vi "Remove Value.vi"(8 "error in (no error)":errorcluster, 10 "Name":string, 11 "Session in":refnum<class "Session.lvclass">) -> (0 "error out":errorcluster, 1 "Found?":bool, 2 "Removed Value":string, 3 "Session out":refnum<class "Session.lvclass">)   [LabVIEW 2020, in "HTTP Server.lvlib" / "Session.lvclass"]
uses:
  Session.lvclass
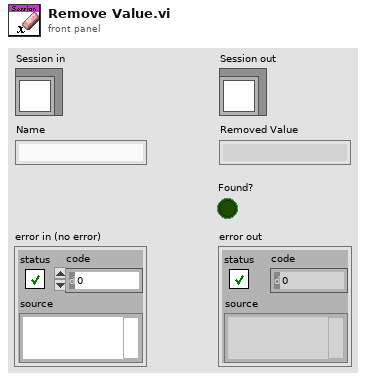
[diagram p1: front panel]
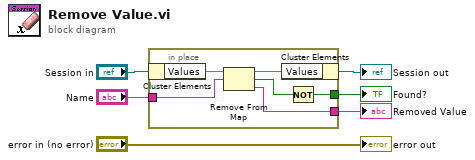
[diagram p0: block diagram]
diagram:
  n1 = in-place {
    in-place-border: "Name" -> [w10]
    in-place-border: [w7] -> w3
    in-place-border: [w8] -> w2
    n2 = in-place-cluster #1("Session in") -> ("Values"=w9:map{string, string})
    n3 = Remove From Map(10:w10, 11:w9) -> (1:w8:string, 2:w11:bool, 3:w12:map{string, string})
    n4 = in-place-cluster #1("Values"=w12) -> (→"Session out":refnum<class "Session.lvclass">)
    n5 = Not(x=w11) -> (.not. x?=w7:bool)
  }
  "Removed Value" <- w2
  "Found?" <- w3
  "error out" <- "error in (no error)"
